vi "Monitor.vi"(1 "User Name":string) -> (0 "Historic Data":T3)   [LabVIEW 2024]
uses:
  controls/Menu_States.ctl
panel:
  out "Heater":enum16{"Off", "Medium", "Maximum"}(ring)
  out "Temp. Display":T1(graph)
  out "Heater Lebel [V]":dbl
  in  "User Control":T2 {"Temp. Min" step=0.1; "Temp. Max" step=0.1}
  out "Temp [ºC]":dbl(slide) scale=0.0..100.0
  out "Ventilator":bool
  in  "Start Acq":bool=TRUE
  in  "Quit":bool
  in  "Stop Acq":bool
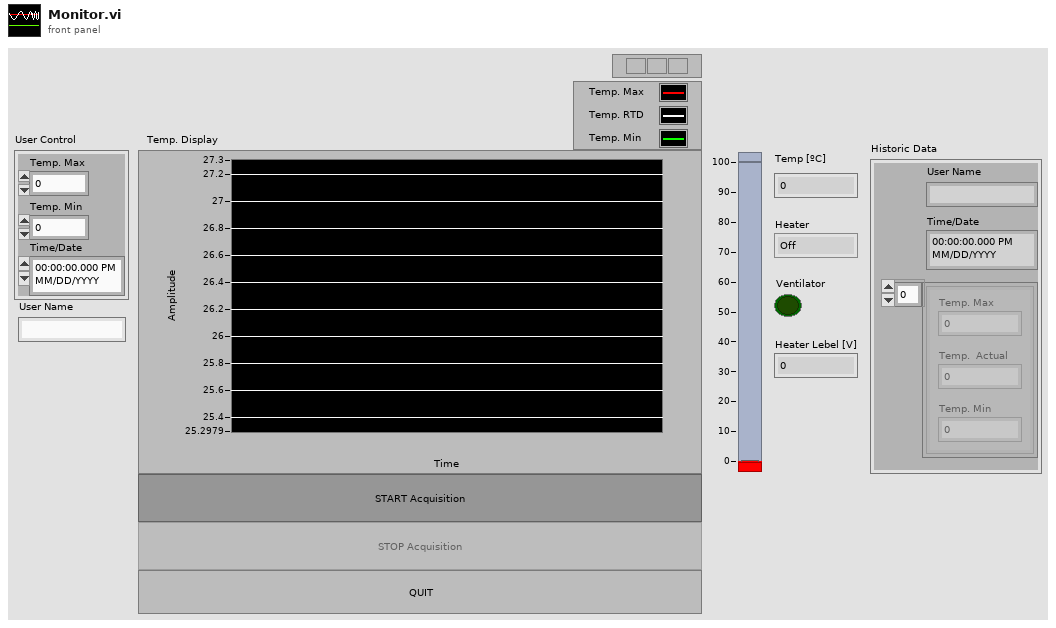
[diagram p1: front panel]
types:
  T1 = cluster{"Temp. Max":dbl, "Temp. Min":dbl, "RTD Temp":dbl}
  T2 = cluster{"Temp. Max":dbl, "Temp. Min":dbl, "Time/Date":timestamp}
  T3 = cluster{"User Name":string, "Time/Date":timestamp, "Array":cluster{"Temp. Max":dbl, "Temp.  Actual":dbl, "Temp. Min":dbl}[]}
  T4 = cluster{"Temp. Max":dbl, "RTD Temp":dbl, "Temp. Min":dbl}[]
  T5 = typedef "Menu_States.ctl" = enum8{"Initialize", "Measure", "Cooling", "Maximum", "Medium", "View Acquired Data", "Quit"}
  T6 = enum8{"Enabled", "Disabled", "Disabled and Grayed Out"}
  T7 = cluster{"Temp. Max":dbl, "Temp. Min":dbl, "RTD Temp":dbl}[]
  T8 = cluster{"Temp. Max":dbl, "RTD Temp":dbl, "Temp. Min":dbl}
  T9 = cluster{"User Name":string, "Time/Date":timestamp, cluster{"Temp. Max":dbl, "RTD Temp":dbl, "Temp. Min":dbl}[]}
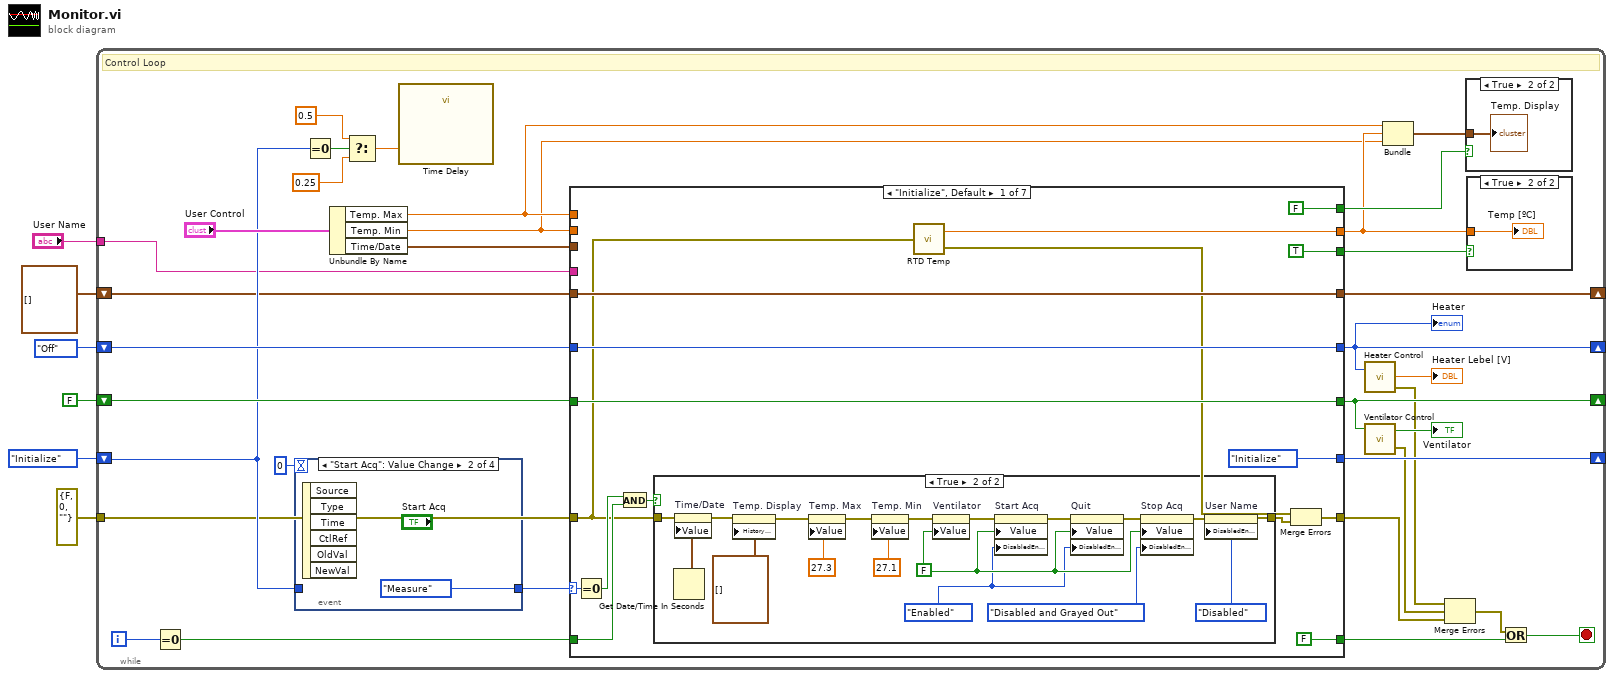
[diagram p0: block diagram]
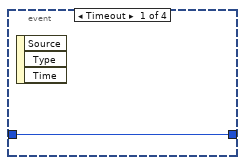
[diagram p3: hidden frame]
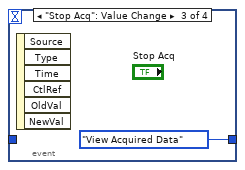
[diagram p4: hidden frame]
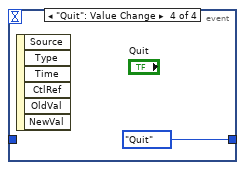
[diagram p5: hidden frame]
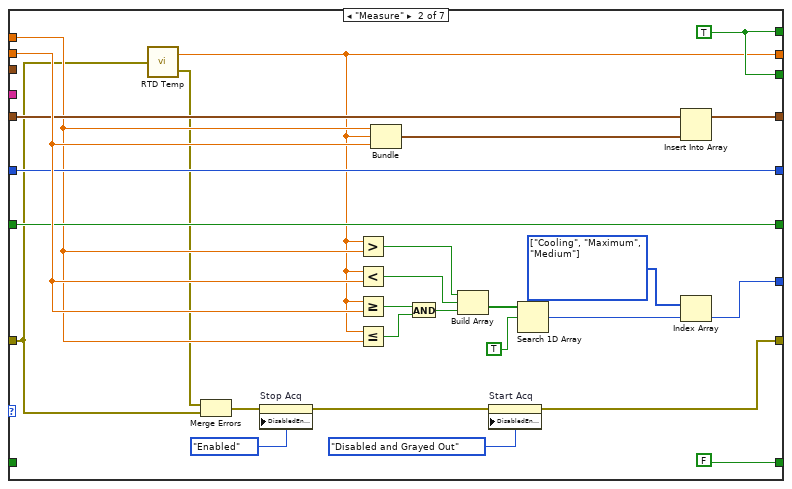
[diagram p8: hidden frame]
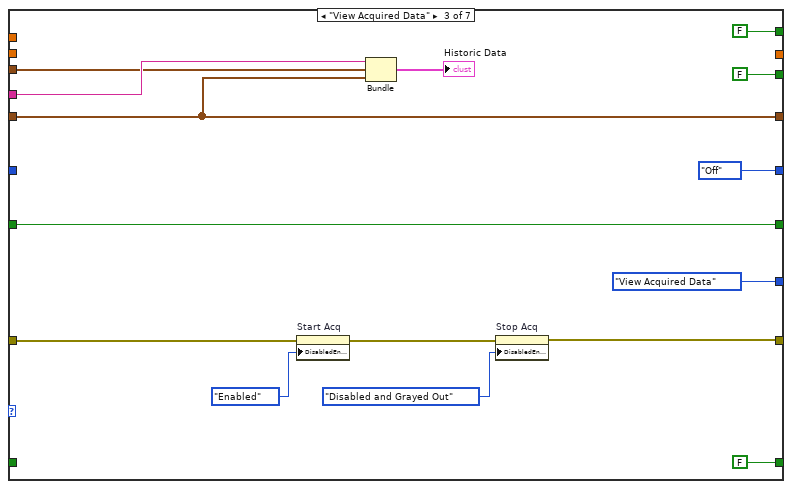
[diagram p9: hidden frame]
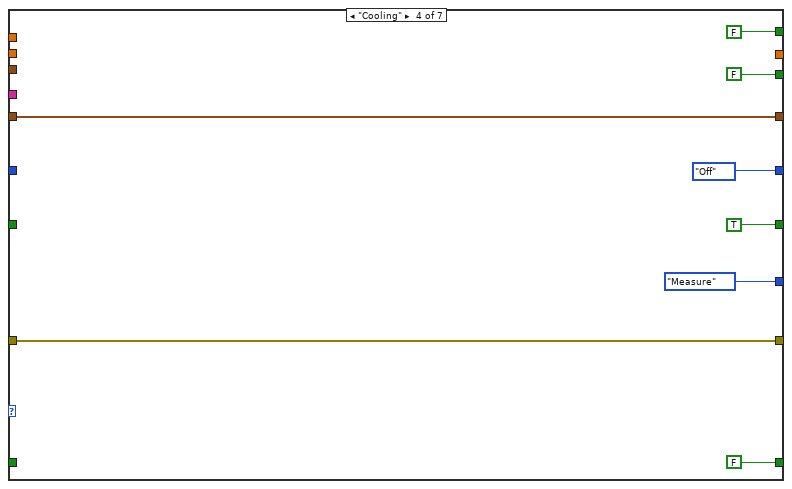
[diagram p10: hidden frame]
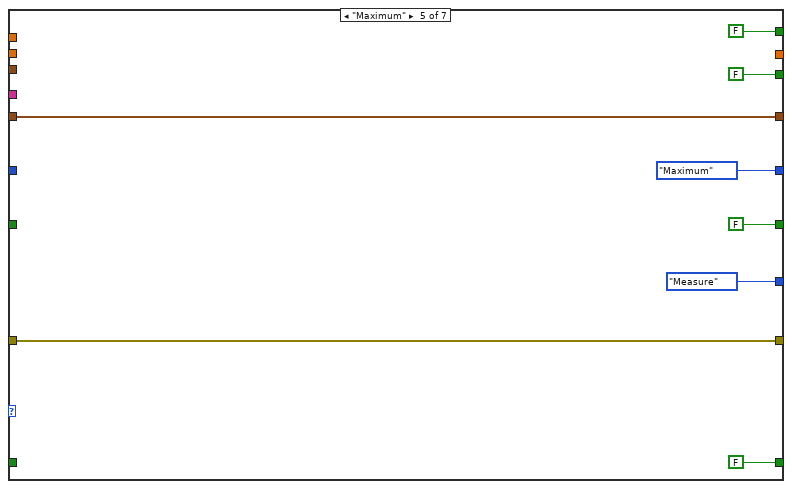
[diagram p11: hidden frame]
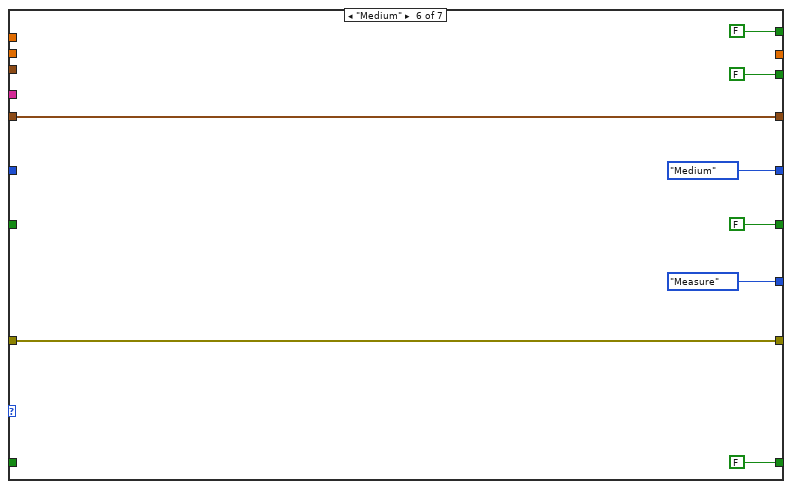
[diagram p12: hidden frame]
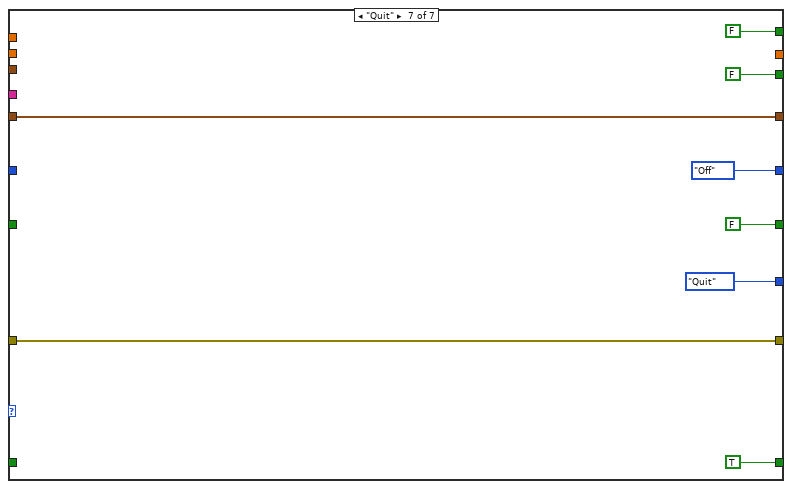
[diagram p13: hidden frame]
diagram:
  n1 = while {
    shift-right: [w36] -> _
    shift-left: Menu_States."Initialize" ("Enum") -> [w24]
    shift-right: [w34] -> _
    shift-left: enum16{"Off", "Medium", "Maximum"}."Off" ("Heater Level") -> [w35]
    shift-right: [w33] -> _
    shift-left: FALSE ("Ventilator (off)") -> [w32]
    shift-right: [w19] -> _
    shift-left: T4 [] -> [w18]
    tunnel: errorcluster {"status"=FALSE, "code"=0, "source"=""} ("error in (no error)") -> [w17]
    tunnel: "User Name" -> [w13]
    i -> [w28]
    stop <- w11 stop-if-true
    # "Control Loop"
    n2 = Equal To 0?(x=w28) -> (x = 0?=w27:bool)
    n3 = event shown="[1] \"Start Acq\": Value Change" {
      selector: _ -> [_ _ _ _]
      dyn-events: _ -> [_ _ _ _]
      timeout: 0 -> [_ _ _ _]
      tunnel: [w42 Menu_States."Measure" ("Enum") Menu_States."View Acquired Data" ("Enum") Menu_States."Quit" ("Enum")] -> w31
      tunnel: w24 -> [w42 _ _ _]
      event Timeout {
        n4 = event-data() -> ()  [unwired: 1 in, 3 out]
      }
      event "Start Acq": Value Change {
        n5 = event-data() -> ()  [unwired: 1 in, 6 out]
      }
      event "Stop Acq": Value Change {
        n6 = event-data() -> ()  [unwired: 1 in, 6 out]
      }
      event "Quit": Value Change {
        n7 = event-data() -> ()  [unwired: 1 in, 6 out]
      }
    }
    n8 = Equal To 0?(x=w24) -> (x = 0?=w23:bool)
    n9 = Unbundle By Name("User Control") -> ("Temp. Max"=w38:dbl, "Temp. Min"=w14:dbl, "Time/Date"=w20:timestamp)
    n10 = Select(t=0.5 ("Delay Time (s)"), s=w23, f=0.25) -> (s? t:f=w22:dbl)
    n11 = call "Time Delay"("Delay Time (s)"=w22) -> ()  [unwired: 10 in, 1 out]
    n12 = case shown="\"Initialize\", Default" w31 {
      selector: w31 -> [w62 _ _ _ _ _ _]
      tunnel: [FALSE FALSE FALSE FALSE FALSE FALSE TRUE] -> w12
      tunnel: w38 -> [_ w86 _ _ _ _ _]
      tunnel: w14 -> [_ w94 _ _ _ _ _]
      tunnel: [Menu_States."Initialize" ("Enum") w98 Menu_States."View Acquired Data" ("Enum") Menu_States."Measure" ("Enum") Menu_States."Measure" ("Enum") Menu_States."Measure" ("Enum") Menu_States."Quit" ("Enum")] -> w36
      tunnel: [FALSE w95 FALSE FALSE FALSE FALSE FALSE] -> w29
      tunnel: w35 -> [w56 w87 _ _ _ _ _]
      tunnel: [w56 w87 enum16{"Off", "Medium", "Maximum"}."Off" ("Heater Level") enum16{"Off", "Medium", "Maximum"}."Off" ("Heater Level") enum16{"Off", "Medium", "Maximum"}."Maximum" ("Heater Level") enum16{"Off", "Medium", "Maximum"}."Medium" ("Heater Level") enum16{"Off", "Medium", "Maximum"}."Off" ("Heater Level")] -> w34
      tunnel: [w55 w88 w117 TRUE ("Ventilator (off)") FALSE ("Ventilator (off)") FALSE ("Ventilator (off)") FALSE ("Ventilator (off)")] -> w33
      tunnel: w32 -> [w55 w88 w117 _ _ _ _]
      tunnel: [w53 w85 _ _ _ _ _] -> w15
      tunnel: [TRUE w95 FALSE FALSE FALSE FALSE FALSE] -> w30
      tunnel: w27 -> [w54 _ _ _ _ _ _]
      tunnel: w13 -> [_ _ w115 _ _ _ _]
      tunnel: w20 -> [_ _ w114 _ _ _ _]
      tunnel: [w51 w92 w112 w125 w134 w141 w149] -> w19
      tunnel: w18 -> [w51 w91 w112 w125 w134 w141 w149]
      tunnel: [w49 w90 w110 w124 w132 w140 w148] -> w7
      tunnel: w17 -> [w47 w83 w109 w124 w132 w140 w148]
      frame "Initialize", Default {
        n13 = Equal To 0?(x=w62) -> (x = 0?=w61:bool)
        n14 = And(x=w61, y=w54) -> (x .and. y?=w60:bool)
        n15 = case shown="True" w60 {
          tunnel: [w63 w65] -> w48
          tunnel: w47 -> [w63 w72]
          frame False {
          }
          frame True {
            w71 = T6."Enabled" ("Disabled")
            w73 = FALSE ("Ventilator")
            n16 = Get Date/Time In Seconds() -> (seconds since 1Jan1904=w81:timestamp)
            n17 = property on="Time/Date" class="AbsTime (strict)"(error in=w72, "Value"=w81) -> (error out=w70:errorcluster)  [unwired: 1 in, 1 out]
            n18 = property on="Temp. Display" class="WFChart (strict)"(error in=w70, "History Data"=T7 []) -> (error out=w69:errorcluster)  [unwired: 1 in, 1 out]
            n19 = property on="Temp. Max" class="DigNum (strict)"(error in=w69, "Value"=27.3) -> (error out=w79:errorcluster)  [unwired: 1 in, 1 out]
            n20 = property on="Temp. Min" class="DigNum (strict)"(error in=w79, "Value"=27.1) -> (error out=w78:errorcluster)  [unwired: 1 in, 1 out]
            n21 = property on="Ventilator" class="Bool (strict)"(error in=w78, "Value"=w73) -> (error out=w77:errorcluster)  [unwired: 1 in, 1 out]
            n22 = property on="Start Acq" class="Bool (strict)"(error in=w77, "Value"=w73, "DisabledEnum"=w71) -> (error out=w76:errorcluster)  [unwired: 1 in, 1 out]
            n23 = property on="Quit" class="Bool (strict)"(error in=w76, "Value"=w73, "DisabledEnum"=w71) -> (error out=w75:errorcluster)  [unwired: 1 in, 1 out]
            n24 = property on="Stop Acq" class="Bool (strict)"(error in=w75, "Value"=w73, "DisabledEnum"=T6."Disabled and Grayed Out" ("Disabled")) -> (error out=w66:errorcluster)  [unwired: 1 in, 1 out]
            n25 = property on="User Name" class="Str"(error in=w66, "DisabledEnum"=T6."Disabled" ("Disabled")) -> (error out=w65:errorcluster)  [unwired: 1 in, 1 out]
          }
        }
        n26 = call "RTD Temp.vi"("error in (no error)"=w47) -> ("RTD Temp"=w53:dbl, "error out"=w50:errorcluster)
        n27 = Merge Errors(w50, w48) -> (w49:errorcluster)
      }
      frame "Measure" {
        w95 = TRUE
        w99 = T5[] [enum."Cooling", enum."Maximum", enum."Medium"] items=["Initialize", "Measure", "Cooling", "Maximum", "Medium", "View Acquired Data", "Quit"] ("array")
        n28 = call "RTD Temp.vi"("error in (no error)"=w83) -> ("RTD Temp"=w85:dbl, "error out"=w84:errorcluster)
        n29 = Merge Errors(w84, w83) -> (w82:errorcluster)
        n30 = property on="Stop Acq" class="Bool (strict)"(error in=w82, "DisabledEnum"=T6."Enabled" ("Disabled")) -> (error out=w89:errorcluster)  [unwired: 1 in, 1 out]
        n31 = Greater?(x=w85, y=w86) -> (0:w96:bool)
        n32 = Less?(x=w85, y=w94) -> (x < y?=w103:bool)
        n33 = Greater Or Equal?(x=w85, y=w94) -> (x >= y?=w102:bool)
        n34 = Less Or Equal?(x=w85, y=w86) -> (x <= y?=w101:bool)
        n35 = Bundle("Temp. Max"=w86, "RTD Temp"=w85, "Temp. Min"=w94) -> (w93:T8)  [unwired: 1 in]
        n36 = And(x=w102, y=w101) -> (x .and. y?=w100:bool)
        n37 = Build Array(w96, w103, w100) -> (w105:bool[])
        n38 = property on="Start Acq" class="Bool (strict)"(error in=w89, "DisabledEnum"=T6."Disabled and Grayed Out" ("Disabled")) -> (error out=w90:errorcluster)  [unwired: 1 in, 1 out]
        n39 = Search 1D Array(1D array=w105, element=TRUE) -> (index of element=w97:i32)  [unwired: 1 in]
        n40 = Insert Into Array(array=w91, new element=w93) -> (w92:T4)  [unwired: 1 in]
        n41 = Index Array(array=w99, index=w97) -> (element=w98:T5)
      }
      frame "View Acquired Data" {
        n42 = property on="Start Acq" class="Bool (strict)"(error in=w109, "DisabledEnum"=T6."Enabled" ("Disabled")) -> (error out=w123:errorcluster)  [unwired: 1 in, 1 out]
        n43 = Bundle("User Name"=w115, "Time/Date"=w114, w112) -> (→"Historic Data":T9)  [unwired: 1 in]
        n44 = property on="Stop Acq" class="Bool (strict)"(error in=w123, "DisabledEnum"=T6."Disabled and Grayed Out" ("Disabled")) -> (error out=w110:errorcluster)  [unwired: 1 in, 1 out]
      }
      frame "Cooling" {
      }
      frame "Maximum" {
      }
      frame "Medium" {
      }
      frame "Quit" {
      }
    }
    "Heater" <- w34
    n45 = call "Heater Control.vi"("Heater Level"=w34) -> ("Heater Level (V)"=→"Heater Lebel [V]":dbl, "error out"=w10:errorcluster)  [unwired: 2 in]
    n46 = call "Ventilator Control.vi"("Ventilator (off)"=w33) -> ("error out"=w9:errorcluster, "Ventilator State"=→"Ventilator":bool)  [unwired: 1 in]
    n47 = Bundle("Temp. Max"=w38, "RTD Temp"=w15, "Temp. Min"=w14) -> (w21:T8)  [unwired: 1 in]
    n48 = Merge Errors(w10, w9, w7) -> (w8:errorcluster)
    n49 = case shown="True" w29 {
      tunnel: w21 -> [_ w46]
      frame False {
      }
      frame True {
        "Temp. Display" <- w46
      }
    }
    n50 = case shown="True" w30 {
      tunnel: w15 -> [_ w41]
      frame False {
      }
      frame True {
        "Temp [ºC]" <- w41
      }
    }
    n51 = Or(x=w8, y=w12) -> (x .or. y?=w11:bool)
  }
